vi "WaveformDataArray.vi"(0 "Max Waveform Size":i32, 5 "Sample Rate":dbl, 9 "Transient":T1={"t1 (ms)"=10.0, "t2 (ms)"=10.0, "t3 (ms)"=10.0, "High Load (A)"=1.0, "Low Load (A)"=0.0, "Slew rate A/us"=0.001}, 11 "error in":errorcluster) -> (4 "Waveform Graph 2":waveform(dbl)(graph), 6 "Total time (ms)":dbl, 15 "error out":errorcluster)   [LabVIEW 2020]
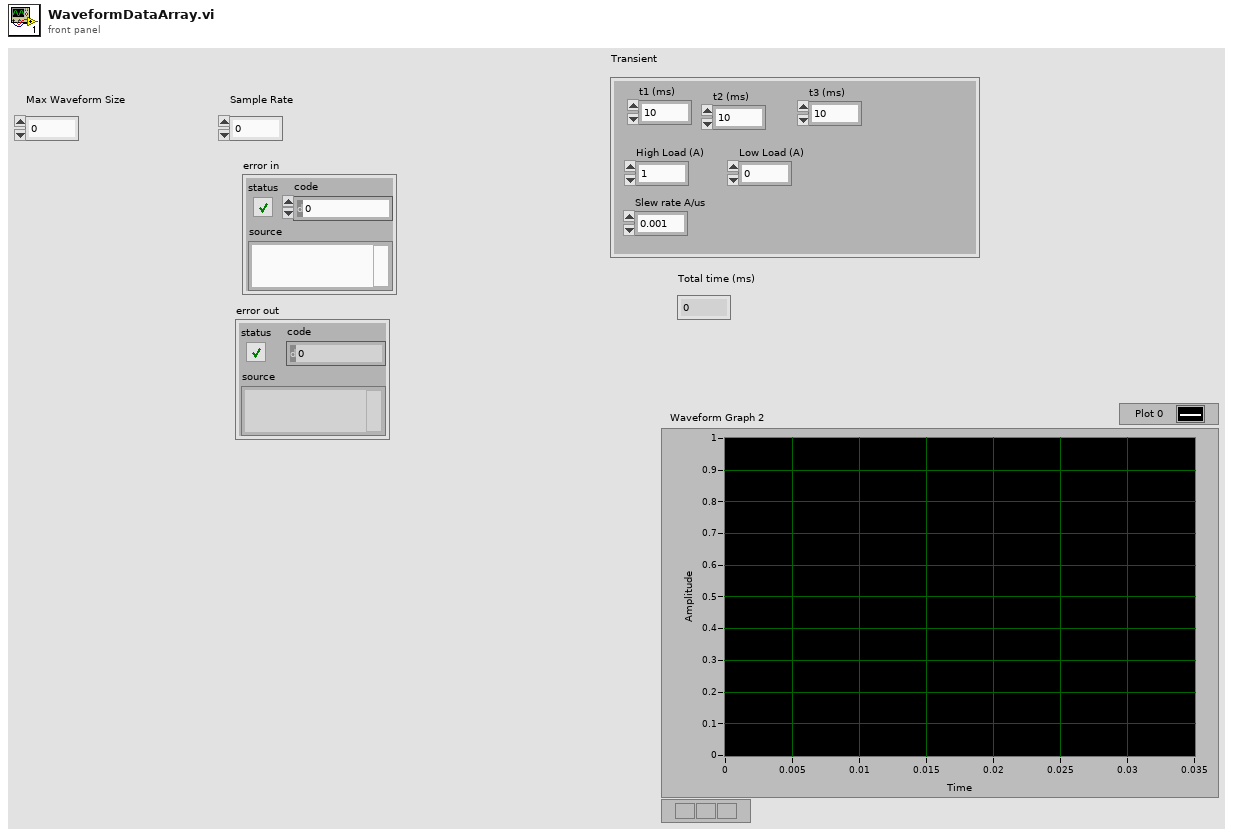
[diagram p1: front panel]
types:
  T1 = cluster{"t1 (ms)":dbl, "t2 (ms)":dbl, "t3 (ms)":dbl, "High Load (A)":dbl, "Low Load (A)":dbl, "Slew rate A/us":dbl}
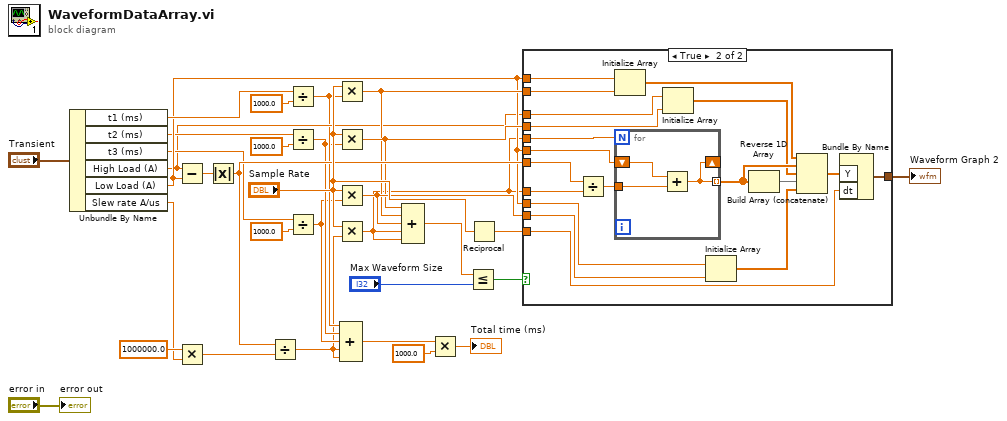
[diagram p0: block diagram]
diagram:
  n1 = Unbundle By Name("Transient") -> ("t1 (ms)"=w13:dbl, "t2 (ms)"=w10:dbl, "t3 (ms)"=w11:dbl, "High Load (A)"=w9:dbl, "Low Load (A)"=w12:dbl, "Slew rate A/us"=w14:dbl)
  n2 = Subtract(x=w9, y=w12) -> (x-y=w26:dbl)
  n3 = Multiply(x=1000000.0, y=w14) -> (x*y=w25:dbl)
  n4 = Absolute Value(x=w26) -> (abs(x)=w22:dbl)
  n5 = Divide(x=w22, y=w25) -> (x/y=w4:dbl)
  n6 = Divide(x=w13, y=1000.0) -> (x/y=w7:dbl)
  n7 = Divide(x=w10, y=1000.0) -> (x/y=w6:dbl)
  n8 = Divide(x=w11, y=1000.0) -> (x/y=w5:dbl)
  n9 = Multiply(x="Sample Rate", y=w7) -> (x*y=w19:dbl)
  n10 = Multiply(x="Sample Rate", y=w6) -> (x*y=w20:dbl)
  n11 = Multiply(x="Sample Rate", y=w5) -> (x*y=w21:dbl)
  n12 = Multiply(x="Sample Rate", y=w4) -> (x*y=w8:dbl)
  n13 = Compound Arithmetic op=ADD(w7, w6, w5, w4, w4) -> (w3:dbl)
  n14 = Compound Arithmetic op=ADD(w20, w19, w21, w8, w8) -> (w17:dbl)
  n15 = Multiply(x=w3, y=1000.0) -> (x*y=→"Total time (ms)":dbl)
  n16 = Less Or Equal?(x=w17, y="Max Waveform Size") -> (x <= y?=w24:bool)
  n17 = Reciprocal(x="Sample Rate") -> (1/x=w23:dbl)
  n18 = case shown="True" w24 {
    tunnel: w23 -> [_ w45]
    tunnel: w8 -> [_ w44]
    tunnel: w22 -> [_ w43]
    tunnel: w8 -> [_ w42]
    tunnel: w12 -> [_ w41]
    tunnel: w12 -> [_ w40]
    tunnel: w21 -> [_ w39]
    tunnel: w9 -> [_ w38]
    tunnel: w20 -> [_ w37]
    tunnel: w12 -> [_ w36]
    tunnel: w19 -> [_ w35]
    tunnel: [_ w34] -> w18
    frame False {
    }
    frame True {
      n19 = Divide(x=w43, y=w44) -> (x/y=w47:dbl)
      n20 = Initialize Array(w36, w35) -> (w46:dbl[])
      n21 = for {
        N: w42 -> [_]
        tunnel: w47 -> [w53]
        tunnel: [w52] -> w50 mode=indexing
        shift-right: [w52] -> _
        shift-left: w41 -> [w54]
        n22 = Add(x=w54, y=w53) -> (x+y=w52:dbl)
      }
      n23 = Initialize Array(w38, w37) -> (w49:dbl[])
      n24 = Initialize Array(w40, w39) -> (w48:dbl[])
      n25 = Reverse 1D Array(array=w50) -> (reversed array=w51:dbl[])
      n26 = Build Array (concatenate)(w46, w50, w49, w51, w48) -> (w33:dbl[])
      n27 = Bundle By Name("Y"=w33, "dt"=w45) -> (w34:waveform(dbl))  [unwired: 1 in]
    }
  }
  "Waveform Graph 2" <- w18
  "error out" <- "error in"
